vi "PicoScopeospaNearestSampleIntervalStateless.vi"(5 "Enabled array":i16[](array[numeric])=[1, 0, 0, 0, 0, 0, 0, 0, 0, 0], 6 "Device Info":T1={"PICO_DRIVER_VERSION"="", "PICO_USB_VERSION"="", "PICO_HARDWARE_VERSION"="", "PICO_VARIANT_INFO"="", "PICO_BATCH_AND_SERIAL"="", "PICO_CAL_DATE"="", "PICO_KERNEL_VERSION"="", "PICO_DIGITAL_HARDWARE_VERSION"="", "PICO_ANALOGUE_HARDWARE_VERSION"="", "PICO_FIRMWARE_VERSION_1"="", "PICO_FIRMWARE_VERSION_2"="", "PICO_IPP_VERSION"="", "PICO_DRIVER_PATH"="", "PICO_FIRMWARE_VERSION_3"="", "PICO_FRONT_PANEL_FIRMWARE_VERSION"="", "Number of Channels"=4, "MSO"=FALSE}, 7 "Resolution":u32(ring)=10 items=["8-bit"=0, "12-bit"=1, "14-bit"=2, "15-bit"=3, "16-bit"=4, "10-bit"=10], 8 "error in (no error)":errorcluster, 9 "roundFaster":u8=1, 10 "timeIntervalRequested":dbl format="%#6_6p", 11 "handle in":i16) -> (0 "error out":errorcluster, 1 "timebase":u32, 2 "timeIntervalAvailable":dbl format="%#6_6p", 3 "handle out":i16)   [LabVIEW 2024]
doc: "Calls Gettimebase function"
uses:
  psospa.dll
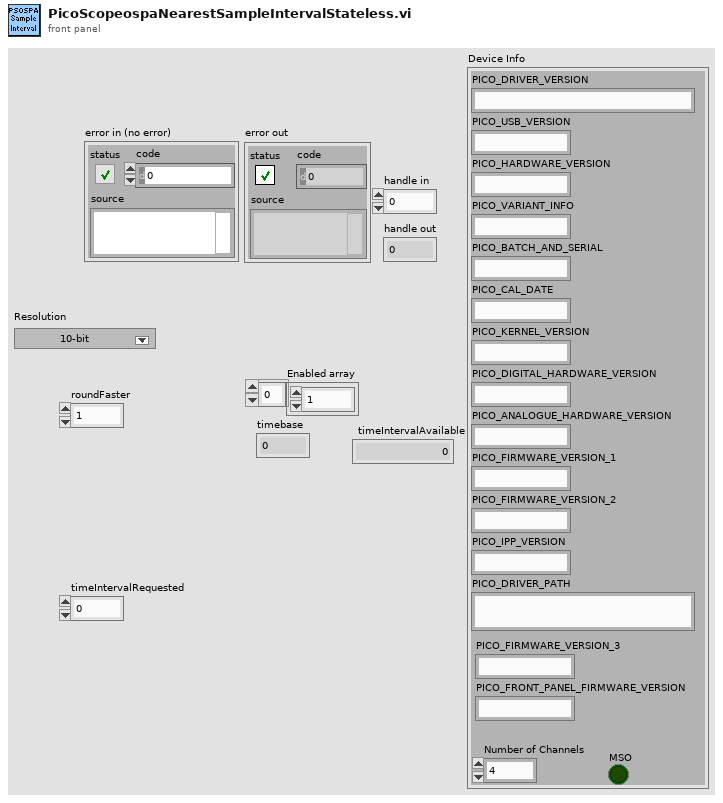
[diagram p1: front panel]
types:
  T1 = cluster{"PICO_DRIVER_VERSION":string, "PICO_USB_VERSION":string, "PICO_HARDWARE_VERSION":string, "PICO_VARIANT_INFO":string, "PICO_BATCH_AND_SERIAL":string, "PICO_CAL_DATE":string, "PICO_KERNEL_VERSION":string, "PICO_DIGITAL_HARDWARE_VERSION":string, "PICO_ANALOGUE_HARDWARE_VERSION":string, "PICO_FIRMWARE_VERSION_1":string, "PICO_FIRMWARE_VERSION_2":string, "PICO_IPP_VERSION":string, "PICO_DRIVER_PATH":string, "PICO_FIRMWARE_VERSION_3":string, "PICO_FRONT_PANEL_FIRMWARE_VERSION":string, "Number of Channels":i16, "MSO":bool}
  T2 = cluster{"status":bool, "code":u32, "source":string}
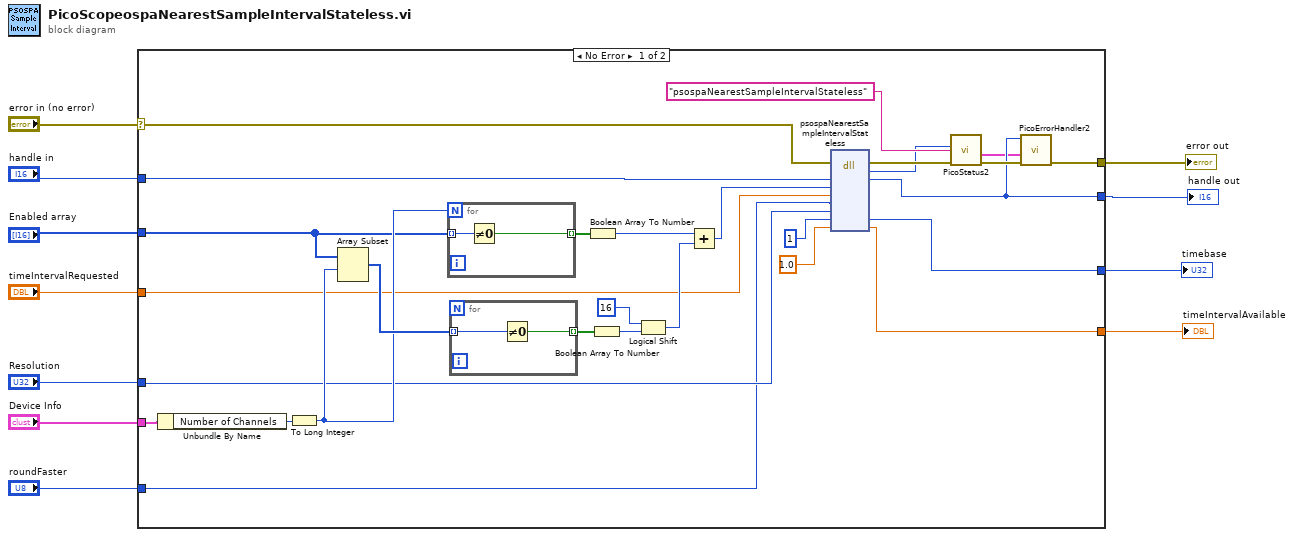
[diagram p0: block diagram]
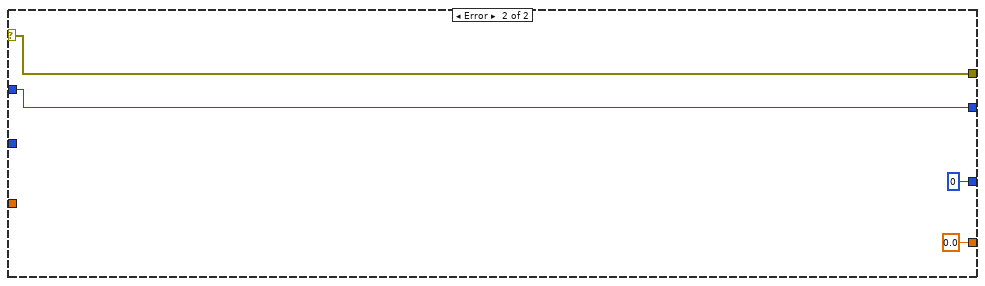
[diagram p2: hidden frame]
diagram:
  n1 = case shown="No Error" "error in (no error)" {
    selector: "error in (no error)" -> [w35 w47]
    tunnel: [w33 w47] -> w11
    tunnel: [w32 w46] -> w10
    tunnel: "handle in" -> [w36 w46]
    tunnel: "Enabled array" -> [w17 _]
    tunnel: "Resolution" -> [w14 _]
    tunnel: "roundFaster" -> [w13 _]
    tunnel: "timeIntervalRequested" -> [w16 _]
    tunnel: [w29 u32 0 ("timebase")] -> w3
    tunnel: [w28 0.0 ("timeIntervalAvailable")] -> w2
    tunnel: "Device Info" -> [w12 _]
    frame No Error {
      n2 = Unbundle By Name(w12) -> ("Number of Channels"=w18:i16)
      n3 = To Long Integer(number=w18) -> (32bit integer=w19:i32)
      n4 = Array Subset(array=w17, index=w19) -> (w25:i16[])  [unwired: 1 in]
      n5 = for {
        N: w19 -> [_]
        tunnel: w17 -> [w43] mode=indexing
        tunnel: [w42] -> w26 mode=indexing
        n6 = Not Equal To 0?(x=w43) -> (x != 0?=w42:bool)
      }
      n7 = for {
        tunnel: w25 -> [w41] mode=indexing
        tunnel: [w40] -> w24 mode=indexing
        n8 = Not Equal To 0?(x=w41) -> (x != 0?=w40:bool)
      }
      n9 = Boolean Array To Number(Boolean array=w26) -> (number=w21:u32)
      n10 = Boolean Array To Number(Boolean array=w24) -> (number=w23:u32)
      n11 = Logical Shift(y=i16 16, x=w23) -> (x << y=w20:u32)
      n12 = Add(x=w21, y=w20) -> (x+y=w15:u32)
      n13 = dll-call lib="F:/Picoscope3000e/Scope_LabView/ps3000e/Treiber_und_SubVis/psospa.dll" fn="psospaNearestSampleIntervalStateless"(error in=w35, "handle"=w36, "enabledChannelFlags"=w15, "timeIntervalRequested"=w16, "roundFaster"=w13, "resolution"=w14, "timebase"=u32 1, "timeIntervalAvailable"=1.0) -> (error out=w39:errorcluster, "PICO_STATUS"=w37:u32, "handle"=w32:i16, "timebase"=w29:u32, "timeIntervalAvailable"=w28:dbl)  [unwired: 6 in, 1 out]
      n14 = call "PicoStatus2.vi"("PICO source"="psospaNearestSampleIntervalStateless" ("source"), "Error in"=w39, "PICO STATUS"=w37) -> ("error out"=w34:errorcluster, "PICO_STATUS out"=w27:T2)  [unwired: 5 in]
      n15 = call "PicoErrorHandler2.vi"("error in (no error)"=w34, "PICO_STATUS in"=w27, "handle In"=w32) -> ("error out"=w33:errorcluster)  [unwired: 8 in]
    }
    frame Error {
    }
  }
  "error out" <- w11
  "handle out" <- w10
  "timebase" <- w3
  "timeIntervalAvailable" <- w2
